vi "TPNT_CloseDevice.vi"(8 "error in (no error)":errorcluster, 11 "Object Refnum In":T1) -> (0 "error out":errorcluster)   [LabVIEW 2016]
uses:
  TPNT_Refnum.ctl
  TPNT_CoreFunction.ctl
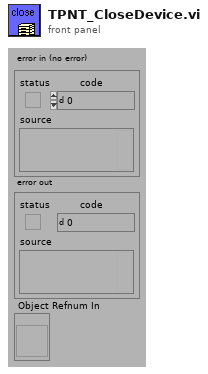
[diagram p1: front panel]
types:
  T1 = typedef "TPNT_Refnum.ctl" = refnum<vi>
  T2 = typedef "TPNT_CoreFunction.ctl" = enum16{"Reset", "Register", "Get Data", "Set Data", "Unregister", "Test", "Get Objects"}
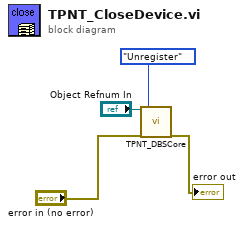
[diagram p0: block diagram]
diagram:
  n1 = call "TPNT_DBSCore.vi"("Object Refnum In"="Object Refnum In", "error in (no error)"="error in (no error)", "Function (Get Data)"=TPNT_CoreFunction."Unregister") -> ("error out"=→"error out":errorcluster)  [unwired: 2 in, 14 out]
